vi "ByPassCom.vi"(8 "error in (no error)":errorcluster, 10 "Param":string, 11 "Controlador in":refnum<class "Controlador.lvclass">) -> (0 "error out":errorcluster, 2 "Resp":string, 3 "Controlador out":refnum<class "Controlador.lvclass">)   [LabVIEW 2012, in "Controlador.lvclass"]
uses:
  Controlador.lvclass
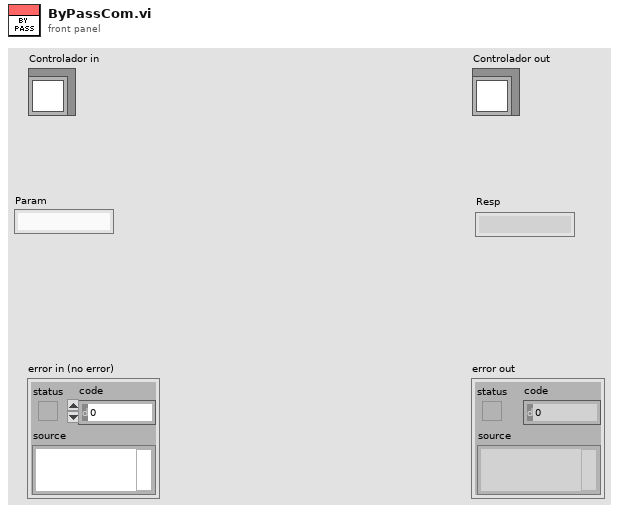
[diagram p1: front panel]
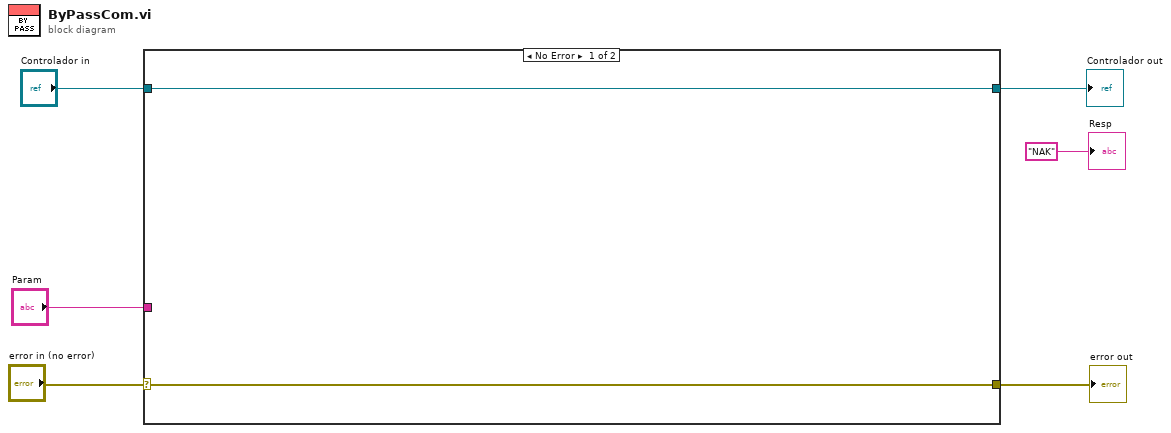
[diagram p0: block diagram]
diagram:
  n1 = case shown="No Error" "error in (no error)" {
    selector: "error in (no error)" -> [w7 w9]
    tunnel: "Controlador in" -> [w8 w10]
    tunnel: [w8 w10] -> w6
    tunnel: [w7 w9] -> w5
    tunnel: "Param" -> [_ _]
    frame No Error {
    }
    frame Error {
    }
  }
  "error out" <- w5
  "Controlador out" <- w6
  "Resp" <- "NAK"
